vi "Test.vi"   [LabVIEW 2019]
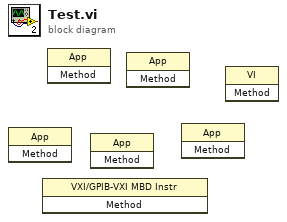
[diagram p0: block diagram]
diagram:
  n1 = invoke class="App" method=#-1() -> ()  [unwired: 3 in, 3 out]
  n2 = invoke class="VXI/GPIB-VXI MBD Instr" method=#-1() -> ()  [unwired: 3 in, 3 out]
  n3 = invoke class="App" method=#-1() -> ()  [unwired: 3 in, 3 out]
  n4 = invoke class="App" method=#-1() -> ()  [unwired: 3 in, 3 out]
  n5 = invoke class="App" method=#-1() -> ()  [unwired: 3 in, 3 out]
  n6 = invoke class="App" method=#-1() -> ()  [unwired: 3 in, 3 out]
  n7 = invoke class="VI" method=#-1() -> ()  [unwired: 3 in, 3 out]
